vi "calculator subvi.vi"(1 "num 5":dbl, 2 "num 6":dbl, 3 "Enum":enum16{"", "add\n", "multiply\n", "subtract\n"}(ring)) -> (0 "result":dbl)   [LabVIEW 2025]
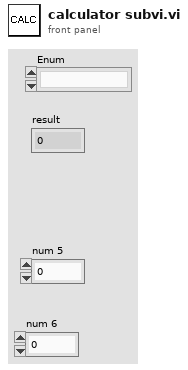
[diagram p1: front panel]
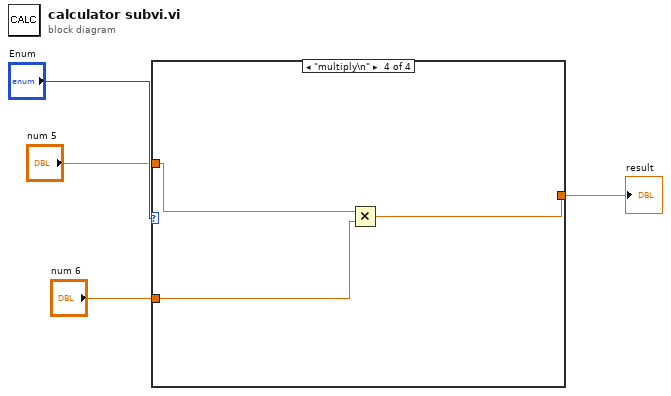
[diagram p0: block diagram]
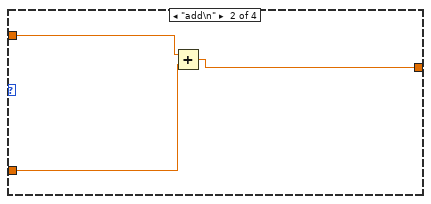
[diagram p3: hidden frame]
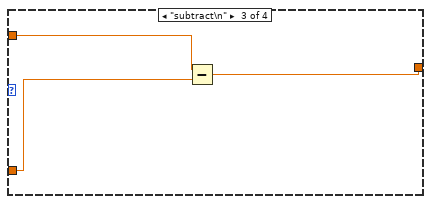
[diagram p4: hidden frame]
diagram:
  n1 = case shown="\"multiply\\n\"" "Enum" {
    tunnel: "num 5" -> [w5 w8 w11 w14]
    tunnel: "num 6" -> [_ w7 w10 w13]
    tunnel: [w5 w6 w9 w12] -> w1
    frame "", Default {
    }
    frame "add\n" {
      n2 = Add(x=w8, y=w7) -> (x+y=w6:dbl)
    }
    frame "subtract\n" {
      n3 = Subtract(x=w11, y=w10) -> (x-y=w9:dbl)
    }
    frame "multiply\n" {
      n4 = Multiply(x=w14, y=w13) -> (x*y=w12:dbl)
    }
  }
  "result" <- w1
